vi "Get Value.vi"(8 "error in (no error)":errorcluster, 11 "Cell in":refnum<class "Cell.lvclass">) -> (0 "error out":errorcluster, 2 "Value":variant, 3 "Cell out":refnum<class "Cell.lvclass">)   [LabVIEW 2024, in "SourceGrid.lvlib" / "Cell.lvclass"]
uses:
  Cell.lvclass
  Cell.lvclass/Cell.ctl
  D:/git/Sourcegrid-LabVIEW/dll/SourceGrid.dll
  dll/SourceGrid.dll
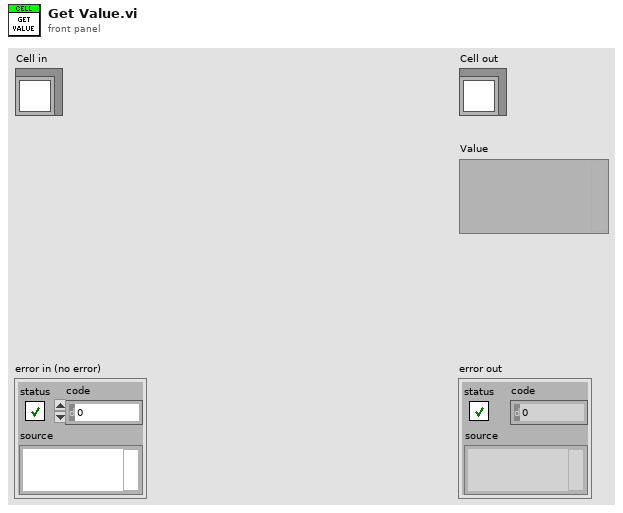
[diagram p1: front panel]
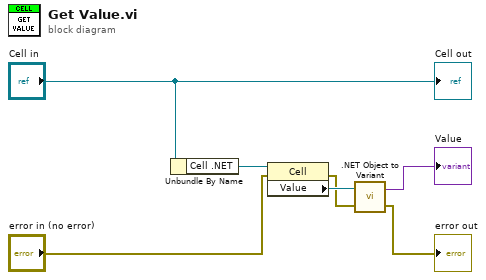
[diagram p0: block diagram]
diagram:
  n1 = Unbundle By Name("Cell in") -> ("Cell .NET"=w5:refnum<k24>)
  n2 = property class="Cell"(reference=w5, error in="error in (no error)") -> (error out=w2:errorcluster, "Value"=w4:refnum<k24>)  [unwired: 1 out]
  n3 = call <vilib>:".NET Object to Variant.vi"("error in (no error)"=w2, ".NET object"=w4) -> ("error out"=→"error out":errorcluster, "variant"=→"Value":variant)
  "Cell out" <- "Cell in"
